vi "BT_Comms_DeBUG_TOOL.vi"() -> ()   [LabVIEW 2016]
panel:
  out "service list":T1(array[cluster])
  out "address out":string
  out "number of services":u16
  out "Numeric":i32
  in  "stop":bool
  out "data out":string
  in  "BT Channel (0)":u16=1
  in  "BT address":string="00:14:03:05:08:37"
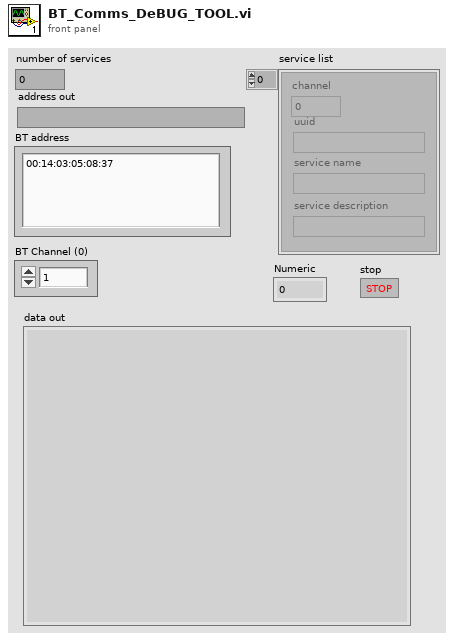
[diagram p1: front panel]
types:
  T1 = cluster{"channel":u16, "uuid":string, "service name":string, "service description":string}[]
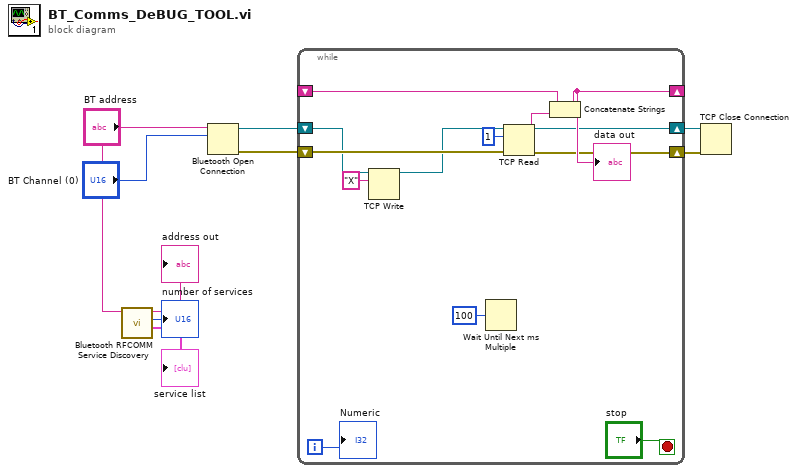
[diagram p0: block diagram]
diagram:
  n1 = call <vilib>:"Bluetooth RFCOMM Service Discovery.vi"("address in"="BT address") -> ("service list"=→"service list":T1, "number of services"=→"number of services":u16, "address out"=→"address out":string)  [unwired: 3 in, 1 out]
  n2 = Bluetooth Open Connection(10:"BT Channel (0)", 11:"BT address") -> (0:w8:errorcluster, 3:w9:refnum<k31>)  [unwired: 3 in]
  n3 = while {
    shift-right: [w15] -> w6
    shift-left: w9 -> [w12]
    shift-right: [w17] -> _
    shift-left: _ -> [w19]
    shift-right: [w16] -> w7
    shift-left: w8 -> [w20]
    i -> [w13]
    stop <- "stop" stop-if-true
    n4 = TCP Write(connection ID=w12, data in="X") -> (connection ID out=w11:refnum<k31>)  [unwired: 2 in, 2 out]
    n5 = Wait Until Next ms Multiple(millisecond multiple=u32 100) -> ()  [unwired: 1 out]
    n6 = TCP Read(connection ID=w11, bytes to read=1, error in (no error)=w20) -> (connection ID out=w15:refnum<k31>, data out=w18:string, error out=w16:errorcluster)  [unwired: 2 in]
    n7 = Concatenate Strings(w19, w18) -> (w17:string)
    "data out" <- w17
    "Numeric" <- w13
  }
  n8 = TCP Close Connection(connection ID=w6, error in (no error)=w7) -> ()  [unwired: 1 in, 2 out]
